vi "main.vi"() -> ()   [LabVIEW 2023]
panel:
  out "Temperature\nOutput":dbl(slide) scale=0.0..100.0
  out "Counter\nIndicator":dbl
  in  "Decrement":bool
  in  "Increment":bool
  # "Display"
  # "Controls"
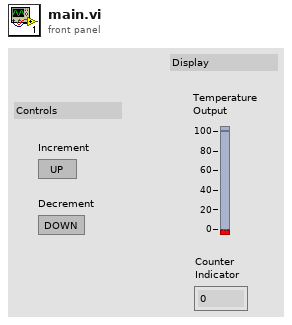
[diagram p1: front panel]
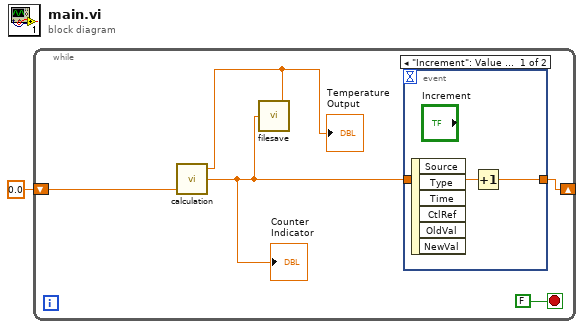
[diagram p0: block diagram]
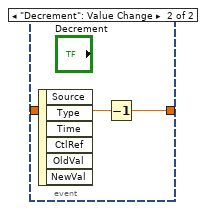
[diagram p2: hidden frame]
diagram:
  n1 = while {
    shift-right: [w5] -> _
    shift-left: 0.0 -> [w4]
    stop <- FALSE stop-if-true
    n2 = call "calculation.vi"("Counter\nInput"=w4) -> ("Counter\nOutput"=w3:dbl, "Temperature\nOutput"=w2:dbl)
    "Counter\nIndicator" <- w3
    "Temperature\nOutput" <- w2
    n3 = call "filesave.vi"("Temperature\nInput"=w2, "Counter\nInput"=w3) -> ()
    n4 = event shown="[0] \"Increment\": Value Change" {
      selector: _ -> [_ _]
      dyn-events: _ -> [_ _]
      timeout: _ -> [_ _]
      tunnel: w3 -> [w8 w10]
      tunnel: [w7 w9] -> w5
      event "Increment": Value Change {
        n5 = event-data() -> ()  [unwired: 1 in, 6 out]
        n6 = Increment(x=w8) -> (x+1=w7:dbl)
      }
      event "Decrement": Value Change {
        n7 = event-data() -> ()  [unwired: 1 in, 6 out]
        n8 = Decrement(x=w10) -> (x-1=w9:dbl)
      }
    }
  }
